vi "PS_EN_ARY.vi"(0 "VISA resource name":refnum<visa-resource-name>, 1 "SEL_PS":string(combo), 11 "error in (no error)":errorcluster {"code" format="%.0x"}, 12 "Enable Output":bool[](array[boolean])) -> (4 "VISA resource name out":refnum<visa-resource-name>, 15 "error out":errorcluster {"code" format="%.0x"})   [LabVIEW 2018]
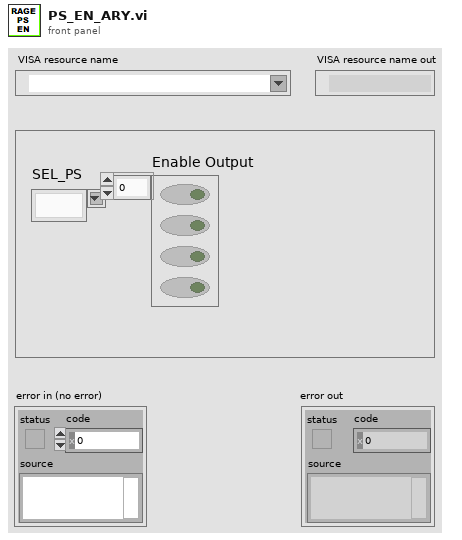
[diagram p1: front panel]
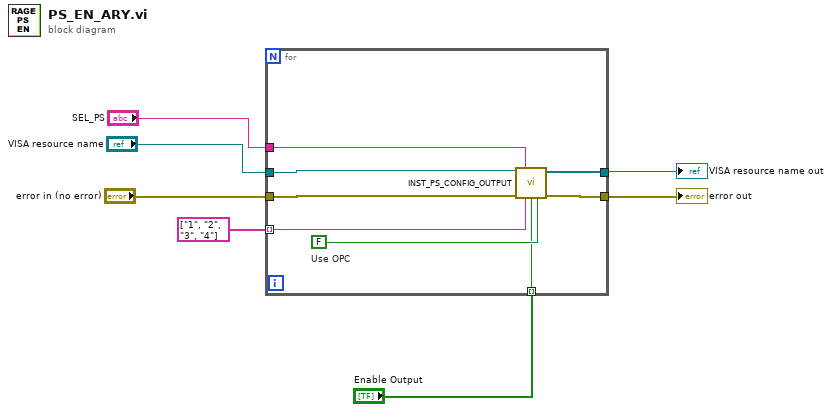
[diagram p0: block diagram]
diagram:
  n1 = for {
    tunnel: string[] ["1", "2", "3", "4"] -> [w15] mode=indexing
    tunnel: "error in (no error)" -> [w14]
    tunnel: [w13] -> w5
    tunnel: "VISA resource name" -> [w12]
    tunnel: [w11] -> w3
    tunnel: "SEL_PS" -> [w10]
    tunnel: "Enable Output" -> [w8] mode=indexing
    w9 = FALSE  # Use OPC
    n2 = call "INST_PS_CONFIG_OUTPUT.vi"("VISA session"=w12, "SEL_PS"=w10, "error in (no error)"=w14, "Instrument Select (Output 1)"=w15, "Enable Output (False)"=w8, "Use OPC(T)"=w9) -> ("dup VISA session"=w11:refnum<visa-resource-name>, "error out"=w13:errorcluster)  [unwired: 7 in, 1 out]
  }
  "error out" <- w5
  "VISA resource name out" <- w3
